vi "auto_calibration.vi"(9 "VISA传感器面板":refnum<visa-resource-name>="COM4", 10 "启动":bool, 11 "VISA灯板":refnum<visa-resource-name>="COM4") -> (3 "进度条":string)   [LabVIEW 2017]
uses:
  <vilib>/LabVIEW Interface for Arduino/Type Defs/Arduino Resource.ctl
  <vilib>/LabVIEW Interface for Arduino/Type Defs/Board Type.ctl
  <vilib>/LabVIEW Interface for Arduino/LabVIEW Interface for Arduino.lvlib
panel:
  out "机电控制报错1":errorcluster
  out "PWM Pins 4":u8[](array[numeric])=[8, 9, 10] caption="PWM Pins 3"
  out "PWM Pins 5":u8[](array[numeric])=[5, 6, 7] caption="PWM Pins 2"
  out "PWM Pins 6":u8[](array[numeric])=[2, 3, 4] caption="PWM Pins"
  out "机电控制资源1":T1={"VISA resource"="", "Board Type"=enum."Uno", "Connection Type"=enum."USB / Serial", "Bytes Per Packet (15)"=15} caption="机电控制资源"
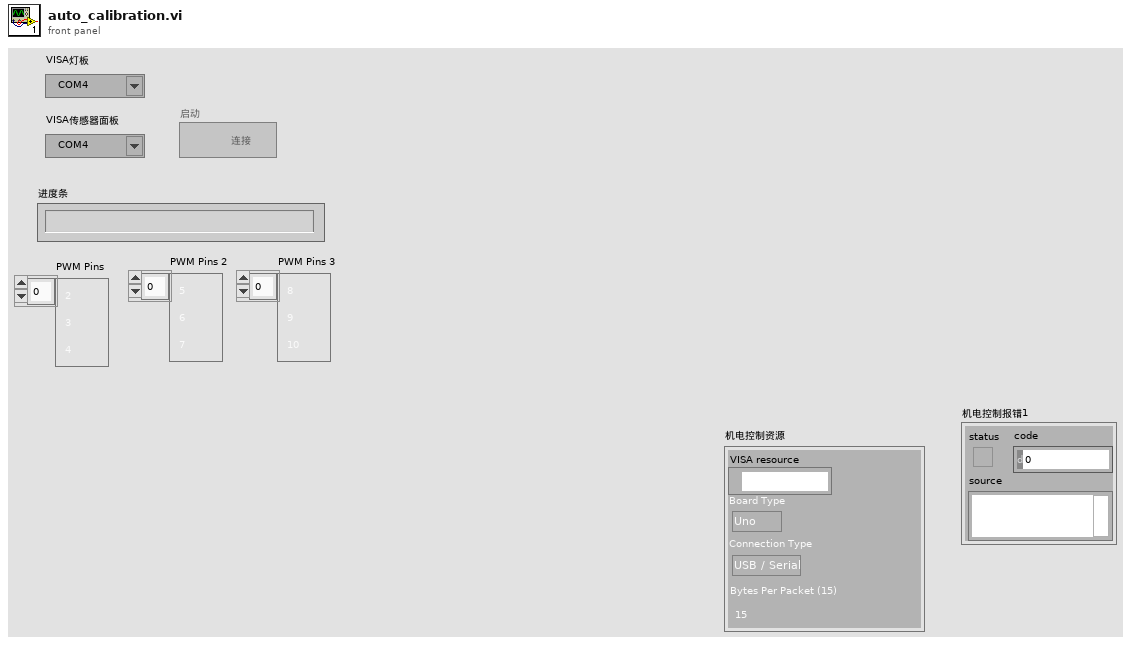
[diagram p1: front panel]
types:
  T1 = typedef "LabVIEW Interface for Arduino.lvlib/Arduino Resource.ctl" = cluster{"VISA resource":refnum<visa-resource-name>, "Board Type":T2, "Connection Type":enum8{"USB / Serial"}, "Bytes Per Packet (15)":u8}
  T2 = typedef "LabVIEW Interface for Arduino.lvlib/Board Type.ctl" = enum16{"Uno", "Dimuelanove w/Atmega 328", "Mega 2560"}
  T3 = enum8{"Enabled", "Disabled", "Disabled and Grayed Out"}
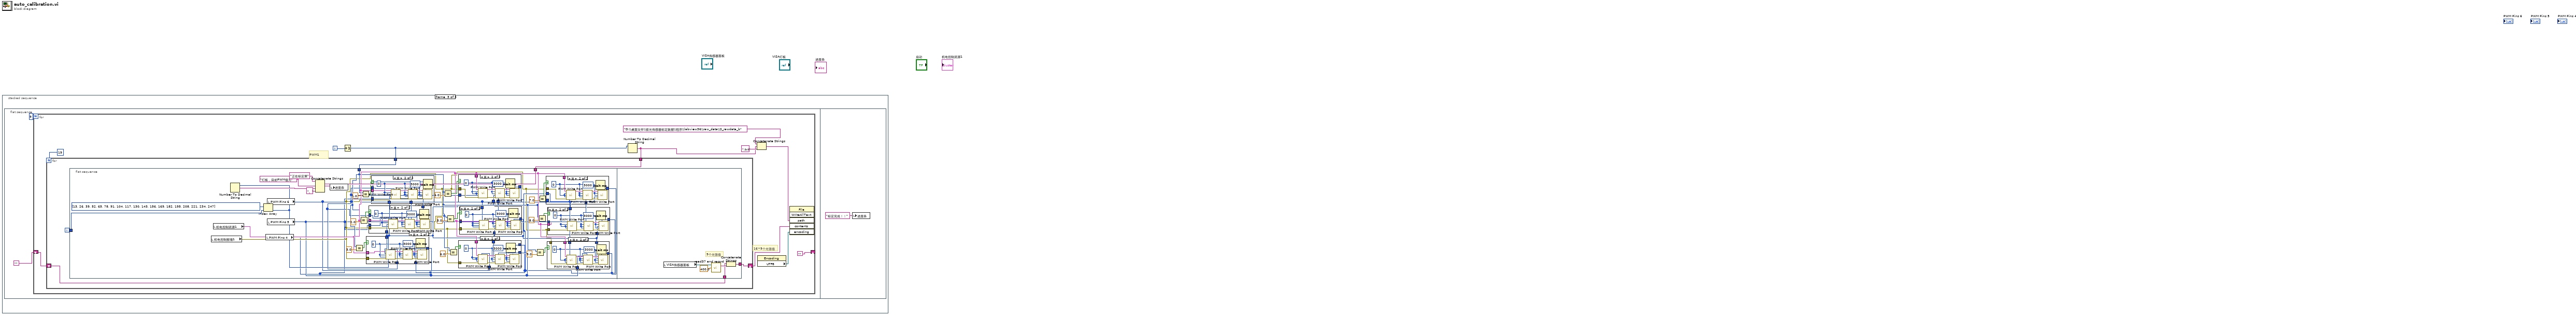
[diagram p0: block diagram]
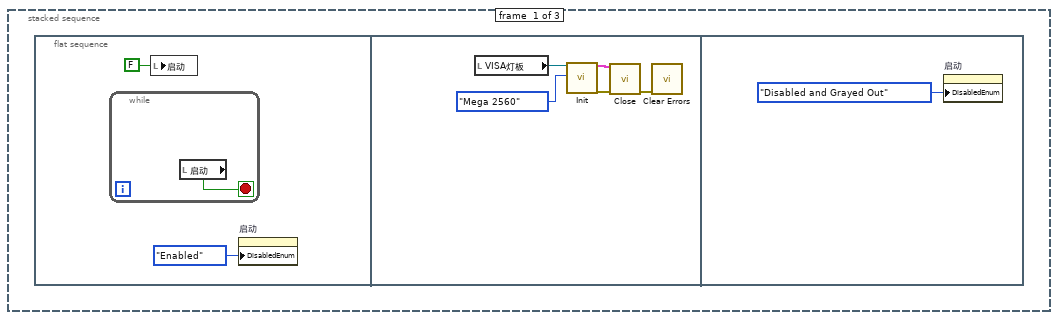
[diagram p2: hidden frame]
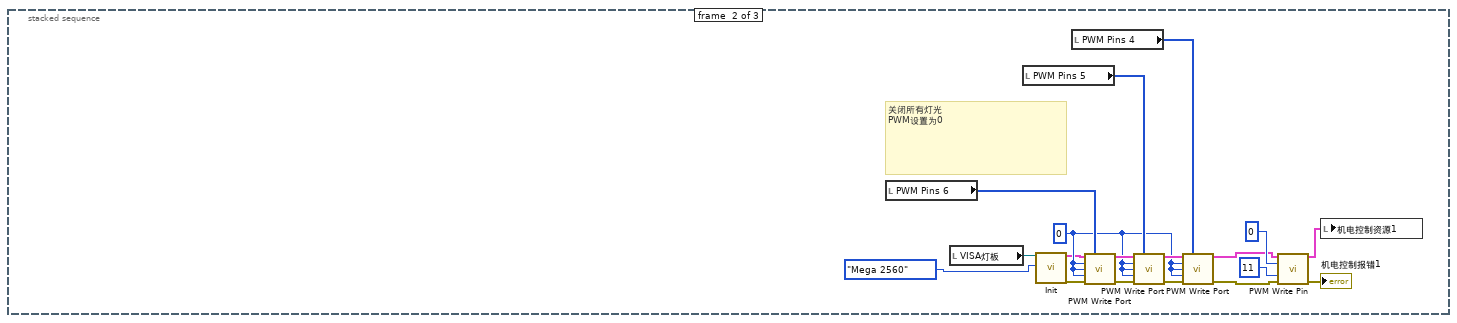
[diagram p3: hidden frame]
diagram:
  n1 = stacked-sequence {
    frame #0 {
      n2 = flat-sequence {
        frame #0 {
          n3 = while {
            stop <- w3 stop-if-true
            n4 = local read "启动"() -> (w3:bool)
          }
          n5 = local write "启动"(FALSE ("启动")) -> ()
          n6 = property on="启动" class="Bool (严格)"("DisabledEnum"=T3."Enabled" ("禁用")) -> ()  [unwired: 2 in, 2 out]
        }
        frame #1 {
          n7 = local read "VISA灯板"() -> (w5:refnum<visa-resource-name>)
          n8 = call <vilib>:"Init.vi"("VISA resource"=w5, "Board Type (Uno)"=Board_Type."Mega 2560") -> ("Arduino Resource"=w8:T1, "error out"=w7:errorcluster)  [unwired: 16 in]
          n9 = call <vilib>:"Close.vi"("Arduino Resource"=w8, "error in"=w7) -> ("error out"=w6:errorcluster)  [unwired: 13 in]
          n10 = call <vilib>:"Clear Errors.vi"("error in (no error)"=w6) -> ()  [unwired: 5 in, 2 out]
        }
        frame #2 {
          n11 = property on="启动" class="Bool (严格)"("DisabledEnum"=T3."Disabled and Grayed Out" ("禁用")) -> ()  [unwired: 2 in, 2 out]
        }
      }
    }
    frame #1 {
      w20 = 0
      # "关闭所有灯光\nPWM设置为0"
      n12 = local read "PWM Pins 6"() -> (w25:u8[])
      n13 = local read "VISA灯板"() -> (w16:refnum<visa-resource-name>)
      n14 = local read "PWM Pins 5"() -> (w26:u8[])
      n15 = call <vilib>:"Init.vi"("VISA resource"=w16, "Board Type (Uno)"=Board_Type."Mega 2560") -> ("Arduino Resource"=w13:T1, "error out"=w14:errorcluster)  [unwired: 16 in]
      n16 = local read "PWM Pins 4"() -> (w27:u8[])
      n17 = call <vilib>:"PWM Write Port.vi"("Arduino Resource"=w13, "PWM Pins"=w25, "PWM 0 (0-255)"=w20, "PWM 1 (0-255)"=w20, "PWM 2 (0-255)"=w20, "error in"=w14) -> ("Arduino Resource"=w21:T1, "error out"=w22:errorcluster)  [unwired: 7 in, 1 out]
      n18 = call <vilib>:"PWM Write Port.vi"("Arduino Resource"=w21, "PWM Pins"=w26, "PWM 0 (0-255)"=w20, "PWM 1 (0-255)"=w20, "PWM 2 (0-255)"=w20, "error in"=w22) -> ("Arduino Resource"=w23:T1, "error out"=w24:errorcluster)  [unwired: 7 in, 1 out]
      n19 = call <vilib>:"PWM Write Port.vi"("Arduino Resource"=w23, "PWM Pins"=w27, "PWM 0 (0-255)"=w20, "PWM 1 (0-255)"=w20, "PWM 2 (0-255)"=w20, "error in"=w24) -> ("Arduino Resource"=w12:T1, "error out"=w11:errorcluster)  [unwired: 7 in, 1 out]
      n20 = call <vilib>:"PWM Write Pin.vi"("Arduino Resource"=w12, "Duty Cycle (0 - 255)"=0, "PWM Pin (3)"=11, "error in"=w11) -> ("Arduino Resource"=w18:T1, "error out"=→"机电控制报错1":errorcluster)  [unwired: 10 in]
      n21 = local write "机电控制资源1"(w18) -> ()
    }
    frame #2 {
      n22 = flat-sequence {
        frame #0 {
          n23 = for {
            N: 9 -> [_]
            shift-right: [""] -> _
            shift-left: "" -> [w31]
            i -> [w36]
            # "16×9个光强值"
            # "PWM1"
            n24 = Increment(x=w36) -> (x+1=w33:i32)
            n25 = Number To Decimal String(number=w33) -> (decimal integer string=w34:string)  [unwired: 1 in]
            n26 = for {
              N: 19 -> [_]
              tunnel: w34 -> [w44]
              tunnel: w33 -> [w43]
              shift-right: [w42] -> w32
              shift-left: w31 -> [w41]
              i -> [w45]
              n27 = flat-sequence {
                tunnel: w45 -> [w77]
                tunnel: w44 -> [w74]
                tunnel: w43 -> [w52]
                tunnel: [w189] -> w42
                tunnel: w41 -> [w187]
                frame #0 {
                  n28 = local read "机电控制报错1"() -> (w49:errorcluster)
                  n29 = local read "机电控制资源1"() -> (w53:T1)
                  n30 = Index Array(array=i32[] [13, 26, 39, 52, 65, 78, 91, 104, 117, 130, 143, 156, 169, 182, 195, 208, 221, 234, 247], index=w77) -> (element=w51:i32)
                  n31 = Number To Decimal String(number=w51) -> (decimal integer string=w75:string)  [unwired: 1 in]
                  n32 = local read "PWM Pins 4"() -> (w46:u8[])
                  n33 = local read "PWM Pins 6"() -> (w48:u8[])
                  n34 = local read "PWM Pins 5"() -> (w47:u8[])
                  n35 = Concatenate Strings("正在标定第" ("进度条"), w74, "灯板，目前PWM值为" ("字符串"), w75, "。" ("字符串")) -> (w76:string)
                  n36 = local write "进度条"(w76) -> ()
                  n37 = Equal?(x=w52, y=3.0) -> (x = y?=w66:bool)
                  n38 = Equal?(x=w52, y=2.0) -> (x = y?=w50:bool)
                  n39 = Equal?(x=w52, y=1.0) -> (x = y?=w70:bool)
                  n40 = case shown="真" w66 {
                    tunnel: w51 -> [_ w157]
                    tunnel: w53 -> [_ w156]
                    tunnel: w49 -> [_ w155]
                    tunnel: w48 -> [_ w154]
                    tunnel: w47 -> [_ w153]
                    tunnel: w46 -> [_ w152]
                    frame False {
                    }
                    frame True {
                      w158 = 0
                      n41 = call <vilib>:"PWM Write Port.vi"("Arduino Resource"=w156, "PWM Pins"=w154, "PWM 0 (0-255)"=w157, "PWM 1 (0-255)"=w158, "PWM 2 (0-255)"=w158, "error in"=w155) -> ("Arduino Resource"=w162:T1, "error out"=w161:errorcluster)  [unwired: 7 in, 1 out]
                      n42 = call <vilib>:"PWM Write Port.vi"("Arduino Resource"=w162, "PWM Pins"=w153, "PWM 0 (0-255)"=w158, "PWM 1 (0-255)"=w158, "PWM 2 (0-255)"=w158, "error in"=w161) -> ("Arduino Resource"=w160:T1, "error out"=w159:errorcluster)  [unwired: 7 in, 1 out]
                      n43 = Wait (ms)(milliseconds to wait=u32 3000 ("等待时间（毫秒）")) -> ()  [unwired: 1 out]
                      n44 = call <vilib>:"PWM Write Port.vi"("Arduino Resource"=w160, "PWM Pins"=w152, "PWM 0 (0-255)"=w158, "PWM 1 (0-255)"=w158, "PWM 2 (0-255)"=w158, "error in"=w159) -> ()  [unwired: 7 in, 3 out]
                    }
                  }
                  n45 = case shown="真" w50 {
                    tunnel: w51 -> [_ w169]
                    tunnel: w53 -> [_ w168]
                    tunnel: w49 -> [_ w167]
                    tunnel: w48 -> [_ w166]
                    tunnel: w47 -> [_ w165]
                    tunnel: w46 -> [_ w164]
                    frame False {
                    }
                    frame True {
                      w170 = 0
                      n46 = call <vilib>:"PWM Write Port.vi"("Arduino Resource"=w168, "PWM Pins"=w166, "PWM 0 (0-255)"=w170, "PWM 1 (0-255)"=w169, "PWM 2 (0-255)"=w170, "error in"=w167) -> ("Arduino Resource"=w174:T1, "error out"=w173:errorcluster)  [unwired: 7 in, 1 out]
                      n47 = call <vilib>:"PWM Write Port.vi"("Arduino Resource"=w174, "PWM Pins"=w165, "PWM 0 (0-255)"=w170, "PWM 1 (0-255)"=w170, "PWM 2 (0-255)"=w170, "error in"=w173) -> ("Arduino Resource"=w172:T1, "error out"=w171:errorcluster)  [unwired: 7 in, 1 out]
                      n48 = Wait (ms)(milliseconds to wait=u32 3000 ("等待时间（毫秒）")) -> ()  [unwired: 1 out]
                      n49 = call <vilib>:"PWM Write Port.vi"("Arduino Resource"=w172, "PWM Pins"=w164, "PWM 0 (0-255)"=w170, "PWM 1 (0-255)"=w170, "PWM 2 (0-255)"=w170, "error in"=w171) -> ()  [unwired: 7 in, 3 out]
                    }
                  }
                  n50 = case shown="真" w70 {
                    tunnel: w53 -> [_ w181]
                    tunnel: w51 -> [_ w180]
                    tunnel: w49 -> [_ w179]
                    tunnel: w48 -> [_ w178]
                    tunnel: w47 -> [_ w177]
                    tunnel: w46 -> [_ w176]
                    frame False {
                    }
                    frame True {
                      w186 = 0
                      n51 = call <vilib>:"PWM Write Port.vi"("Arduino Resource"=w181, "PWM Pins"=w178, "PWM 0 (0-255)"=w186, "PWM 1 (0-255)"=w186, "PWM 2 (0-255)"=w180, "error in"=w179) -> ("Arduino Resource"=w185:T1, "error out"=w184:errorcluster)  [unwired: 7 in, 1 out]
                      n52 = call <vilib>:"PWM Write Port.vi"("Arduino Resource"=w185, "PWM Pins"=w177, "PWM 0 (0-255)"=w186, "PWM 1 (0-255)"=w186, "PWM 2 (0-255)"=w186, "error in"=w184) -> ("Arduino Resource"=w183:T1, "error out"=w182:errorcluster)  [unwired: 7 in, 1 out]
                      n53 = call <vilib>:"PWM Write Port.vi"("Arduino Resource"=w183, "PWM Pins"=w176, "PWM 0 (0-255)"=w186, "PWM 1 (0-255)"=w186, "PWM 2 (0-255)"=w186, "error in"=w182) -> ()  [unwired: 7 in, 3 out]
                      n54 = Wait (ms)(milliseconds to wait=u32 3000 ("等待时间（毫秒）")) -> ()  [unwired: 1 out]
                    }
                  }
                  n55 = Equal?(x=w52, y=4.0) -> (x = y?=w59:bool)
                  n56 = Equal?(x=w52, y=5.0) -> (x = y?=w58:bool)
                  n57 = Equal?(x=w52, y=6.0) -> (x = y?=w57:bool)
                  n58 = case shown="真" w59 {
                    tunnel: w53 -> [_ w146]
                    tunnel: w51 -> [_ w144]
                    tunnel: w49 -> [_ w143]
                    tunnel: w48 -> [_ w142]
                    tunnel: w47 -> [_ w141]
                    tunnel: w46 -> [_ w140]
                    frame False {
                    }
                    frame True {
                      w145 = 0
                      n59 = call <vilib>:"PWM Write Port.vi"("Arduino Resource"=w146, "PWM Pins"=w142, "PWM 0 (0-255)"=w145, "PWM 1 (0-255)"=w145, "PWM 2 (0-255)"=w145, "error in"=w143) -> ("Arduino Resource"=w150:T1, "error out"=w149:errorcluster)  [unwired: 7 in, 1 out]
                      n60 = call <vilib>:"PWM Write Port.vi"("Arduino Resource"=w150, "PWM Pins"=w141, "PWM 0 (0-255)"=w145, "PWM 1 (0-255)"=w145, "PWM 2 (0-255)"=w144, "error in"=w149) -> ("Arduino Resource"=w148:T1, "error out"=w147:errorcluster)  [unwired: 7 in, 1 out]
                      n61 = Wait (ms)(milliseconds to wait=u32 3000 ("等待时间（毫秒）")) -> ()  [unwired: 1 out]
                      n62 = call <vilib>:"PWM Write Port.vi"("Arduino Resource"=w148, "PWM Pins"=w140, "PWM 0 (0-255)"=w145, "PWM 1 (0-255)"=w145, "PWM 2 (0-255)"=w145, "error in"=w147) -> ()  [unwired: 7 in, 3 out]
                    }
                  }
                  n63 = case shown="真" w57 {
                    tunnel: w53 -> [_ w122]
                    tunnel: w51 -> [_ w120]
                    tunnel: w49 -> [_ w119]
                    tunnel: w48 -> [_ w118]
                    tunnel: w47 -> [_ w117]
                    tunnel: w46 -> [_ w116]
                    frame False {
                    }
                    frame True {
                      w121 = 0
                      n64 = call <vilib>:"PWM Write Port.vi"("Arduino Resource"=w122, "PWM Pins"=w118, "PWM 0 (0-255)"=w121, "PWM 1 (0-255)"=w121, "PWM 2 (0-255)"=w121, "error in"=w119) -> ("Arduino Resource"=w126:T1, "error out"=w125:errorcluster)  [unwired: 7 in, 1 out]
                      n65 = call <vilib>:"PWM Write Port.vi"("Arduino Resource"=w126, "PWM Pins"=w117, "PWM 0 (0-255)"=w120, "PWM 1 (0-255)"=w121, "PWM 2 (0-255)"=w121, "error in"=w125) -> ("Arduino Resource"=w124:T1, "error out"=w123:errorcluster)  [unwired: 7 in, 1 out]
                      n66 = Wait (ms)(milliseconds to wait=u32 3000 ("等待时间（毫秒）")) -> ()  [unwired: 1 out]
                      n67 = call <vilib>:"PWM Write Port.vi"("Arduino Resource"=w124, "PWM Pins"=w116, "PWM 0 (0-255)"=w121, "PWM 1 (0-255)"=w121, "PWM 2 (0-255)"=w121, "error in"=w123) -> ()  [unwired: 7 in, 3 out]
                    }
                  }
                  n68 = case shown="真" w58 {
                    tunnel: w53 -> [_ w134]
                    tunnel: w51 -> [_ w132]
                    tunnel: w49 -> [_ w131]
                    tunnel: w48 -> [_ w130]
                    tunnel: w47 -> [_ w129]
                    tunnel: w46 -> [_ w128]
                    frame False {
                    }
                    frame True {
                      w133 = 0
                      n69 = call <vilib>:"PWM Write Port.vi"("Arduino Resource"=w134, "PWM Pins"=w130, "PWM 0 (0-255)"=w133, "PWM 1 (0-255)"=w133, "PWM 2 (0-255)"=w133, "error in"=w131) -> ("Arduino Resource"=w138:T1, "error out"=w137:errorcluster)  [unwired: 7 in, 1 out]
                      n70 = call <vilib>:"PWM Write Port.vi"("Arduino Resource"=w138, "PWM Pins"=w129, "PWM 0 (0-255)"=w133, "PWM 1 (0-255)"=w132, "PWM 2 (0-255)"=w133, "error in"=w137) -> ("Arduino Resource"=w136:T1, "error out"=w135:errorcluster)  [unwired: 7 in, 1 out]
                      n71 = Wait (ms)(milliseconds to wait=u32 3000 ("等待时间（毫秒）")) -> ()  [unwired: 1 out]
                      n72 = call <vilib>:"PWM Write Port.vi"("Arduino Resource"=w136, "PWM Pins"=w128, "PWM 0 (0-255)"=w133, "PWM 1 (0-255)"=w133, "PWM 2 (0-255)"=w133, "error in"=w135) -> ()  [unwired: 7 in, 3 out]
                    }
                  }
                  n73 = Equal?(x=w52, y=9.0) -> (x = y?=w54:bool)
                  n74 = Equal?(x=w52, y=8.0) -> (x = y?=w55:bool)
                  n75 = Equal?(x=w52, y=7.0) -> (x = y?=w56:bool)
                  n76 = case shown="真" w56 {
                    tunnel: w53 -> [_ w110]
                    tunnel: w51 -> [_ w108]
                    tunnel: w49 -> [_ w107]
                    tunnel: w48 -> [_ w106]
                    tunnel: w47 -> [_ w105]
                    tunnel: w46 -> [_ w104]
                    frame False {
                    }
                    frame True {
                      w109 = 0
                      n77 = call <vilib>:"PWM Write Port.vi"("Arduino Resource"=w110, "PWM Pins"=w106, "PWM 0 (0-255)"=w109, "PWM 1 (0-255)"=w109, "PWM 2 (0-255)"=w109, "error in"=w107) -> ("Arduino Resource"=w114:T1, "error out"=w113:errorcluster)  [unwired: 7 in, 1 out]
                      n78 = call <vilib>:"PWM Write Port.vi"("Arduino Resource"=w114, "PWM Pins"=w105, "PWM 0 (0-255)"=w109, "PWM 1 (0-255)"=w109, "PWM 2 (0-255)"=w109, "error in"=w113) -> ("Arduino Resource"=w112:T1, "error out"=w111:errorcluster)  [unwired: 7 in, 1 out]
                      n79 = Wait (ms)(milliseconds to wait=u32 3000 ("等待时间（毫秒）")) -> ()  [unwired: 1 out]
                      n80 = call <vilib>:"PWM Write Port.vi"("Arduino Resource"=w112, "PWM Pins"=w104, "PWM 0 (0-255)"=w109, "PWM 1 (0-255)"=w109, "PWM 2 (0-255)"=w108, "error in"=w111) -> ()  [unwired: 7 in, 3 out]
                    }
                  }
                  n81 = case shown="真" w54 {
                    tunnel: w53 -> [_ w86]
                    tunnel: w51 -> [_ w84]
                    tunnel: w49 -> [_ w83]
                    tunnel: w48 -> [_ w82]
                    tunnel: w47 -> [_ w81]
                    tunnel: w46 -> [_ w80]
                    frame False {
                    }
                    frame True {
                      w85 = 0
                      n82 = call <vilib>:"PWM Write Port.vi"("Arduino Resource"=w86, "PWM Pins"=w82, "PWM 0 (0-255)"=w85, "PWM 1 (0-255)"=w85, "PWM 2 (0-255)"=w85, "error in"=w83) -> ("Arduino Resource"=w90:T1, "error out"=w89:errorcluster)  [unwired: 7 in, 1 out]
                      n83 = call <vilib>:"PWM Write Port.vi"("Arduino Resource"=w90, "PWM Pins"=w81, "PWM 0 (0-255)"=w85, "PWM 1 (0-255)"=w85, "PWM 2 (0-255)"=w85, "error in"=w89) -> ("Arduino Resource"=w88:T1, "error out"=w87:errorcluster)  [unwired: 7 in, 1 out]
                      n84 = Wait (ms)(milliseconds to wait=u32 3000 ("等待时间（毫秒）")) -> ()  [unwired: 1 out]
                      n85 = call <vilib>:"PWM Write Port.vi"("Arduino Resource"=w88, "PWM Pins"=w80, "PWM 0 (0-255)"=w84, "PWM 1 (0-255)"=w85, "PWM 2 (0-255)"=w85, "error in"=w87) -> ()  [unwired: 7 in, 3 out]
                    }
                  }
                  n86 = case shown="真" w55 {
                    tunnel: w53 -> [_ w98]
                    tunnel: w51 -> [_ w96]
                    tunnel: w49 -> [_ w95]
                    tunnel: w48 -> [_ w94]
                    tunnel: w47 -> [_ w93]
                    tunnel: w46 -> [_ w92]
                    frame False {
                    }
                    frame True {
                      w97 = 0
                      n87 = call <vilib>:"PWM Write Port.vi"("Arduino Resource"=w98, "PWM Pins"=w94, "PWM 0 (0-255)"=w97, "PWM 1 (0-255)"=w97, "PWM 2 (0-255)"=w97, "error in"=w95) -> ("Arduino Resource"=w102:T1, "error out"=w101:errorcluster)  [unwired: 7 in, 1 out]
                      n88 = call <vilib>:"PWM Write Port.vi"("Arduino Resource"=w102, "PWM Pins"=w93, "PWM 0 (0-255)"=w97, "PWM 1 (0-255)"=w97, "PWM 2 (0-255)"=w97, "error in"=w101) -> ("Arduino Resource"=w100:T1, "error out"=w99:errorcluster)  [unwired: 7 in, 1 out]
                      n89 = Wait (ms)(milliseconds to wait=u32 3000 ("等待时间（毫秒）")) -> ()  [unwired: 1 out]
                      n90 = call <vilib>:"PWM Write Port.vi"("Arduino Resource"=w100, "PWM Pins"=w92, "PWM 0 (0-255)"=w97, "PWM 1 (0-255)"=w96, "PWM 2 (0-255)"=w97, "error in"=w99) -> ()  [unwired: 7 in, 3 out]
                    }
                  }
                }
                frame #1 {
                  # "9个光强值"
                  n91 = local read "VISA传感器面板"() -> (w191:refnum<visa-resource-name>)
                  n92 = call "read37 and record.vi"("Interval_ms"=400.0, "VISA资源名称"=w191) -> ("本次记录到的字符串"=w188:string)  [unwired: 2 in]
                  n93 = Concatenate Strings(w187, w188) -> (w189:string)
                }
              }
            }
            n94 = Concatenate Strings("D:\\桌面文件\\紫光传感器标定数据\\程序\\labview36\\raw_data\\S_rawdata_b" ("path"), w34, ".txt" ("字符串")) -> (w35:string)
            n95 = property class="Encoding"() -> ("UTF8"=w39:refnum<k24>)  [unwired: 2 in, 2 out]
            n96 = invoke on="调用节点" class="File" method="WriteAllText"("path"=w35, "contents"=w32, "encoding"=w39) -> ()  [unwired: 3 in, 6 out]
          }
        }
        frame #1 {
          n97 = local write "进度条"("标定完成！！" ("进度条")) -> ()
        }
      }
    }
  }
